vi "zmq curve keypair.vi"(8 "error in (no error)":errorcluster, 10 "z85_secret_key_":string, 11 "z85_public_key_":string) -> (0 "error out":errorcluster, 1 "function return":i32, 2 "z85_secret_key_ out":string, 3 "z85_public_key_ out":string)   [LabVIEW 2025, in "libzmq-v143-mt-4_3_6.lvlib"]
doc: "ZMQ_EXPORT int zmq_curve_keypair (char *z85_public_key_, char *z85_secret_key_);"
uses:
  libzmq-v143-mt-4_3_6.lvlib
  LV/LibZMQ/libzmq/lv_x86/bin/Release/libzmq-v143-mt-4_3_6.dll
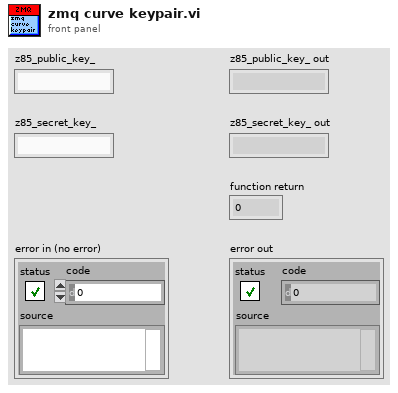
[diagram p1: front panel]
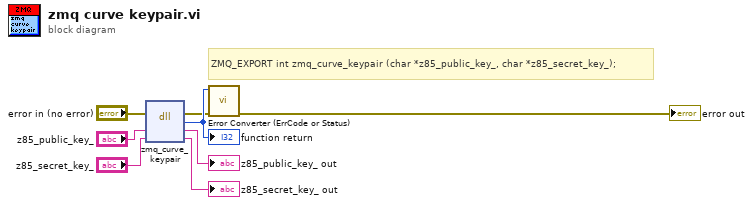
[diagram p0: block diagram]
diagram:
  # "ZMQ_EXPORT int zmq_curve_keypair (char *z85_public_key_, char *z85_secret_key_);"
  n1 = dll-call lib="C:/LV/LibZMQ/libzmq/lv_x86/bin/Release/libzmq-v143-mt-4_3_6.*" fn="zmq_curve_keypair"(error in="error in (no error)", "z85_public_key_"="z85_public_key_", "z85_secret_key_"="z85_secret_key_") -> (error out=w2:errorcluster, w8:i32, "z85_public_key_"=→"z85_public_key_ out":string, "z85_secret_key_"=→"z85_secret_key_ out":string)  [unwired: 2 in, 1 out]
  "function return" <- w8
  n2 = call "Error Converter (ErrCode or Status).vi"("error in (no error)"=w2, "error code"=w8) -> ("error out"=→"error out":errorcluster)  [unwired: 9 in]
